vi "流程固件设置对话框.vi"() -> ()   [LabVIEW 2016, in "斯坦道总磷.lvlib"]
uses:
  <vilib>/Utility/miscctls.llb/LVPointTypeDef.ctl
panel:
  in  "修改系列号":bool
  in  "关闭":bool
  in  "外设设置":bool
  in  "固件升级":bool
  in  "流程写入":bool
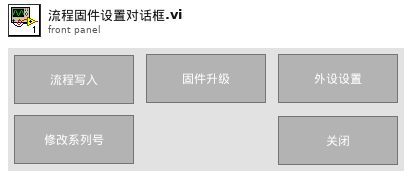
[diagram p1: front panel]
types:
  T1 = typedef "LVPointTypeDef.ctl" = cluster{"Horizontal":i16, "Vertical":i16}
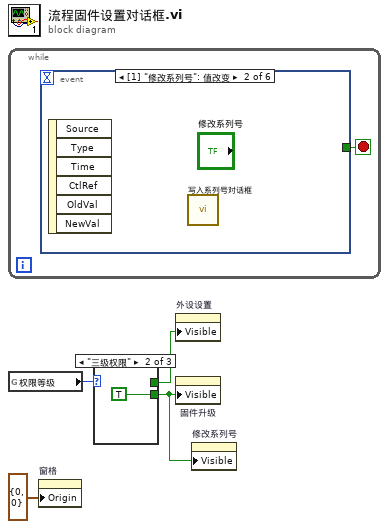
[diagram p0: block diagram]
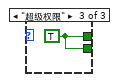
[diagram p3: hidden frame]
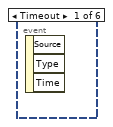
[diagram p4: hidden frame]
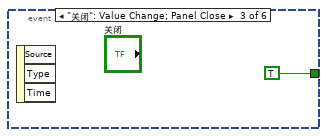
[diagram p5: hidden frame]
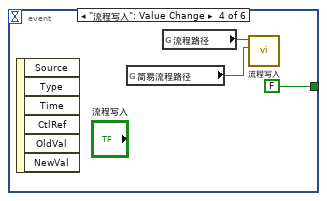
[diagram p6: hidden frame]
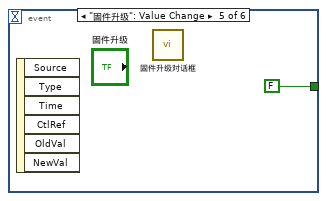
[diagram p7: hidden frame]
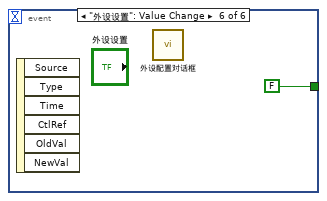
[diagram p8: hidden frame]
diagram:
  n1 = while {
    stop <- w5 stop-if-true
    n2 = event shown="[1] \"修改系列号\": 值改变" {
      selector: _ -> [_ _ _ _ _ _]
      dyn-events: _ -> [_ _ _ _ _ _]
      timeout: _ -> [_ _ _ _ _ _]
      tunnel: [_ _ TRUE FALSE FALSE FALSE] -> w5
      event Timeout {
        n3 = event-data() -> ()  [unwired: 1 in, 3 out]
      }
      event "修改系列号": Value Change {
        n4 = event-data() -> ()  [unwired: 1 in, 6 out]
        n5 = call "写入系列号对话框.vi"() -> ()  [unwired: 12 in]
      }
      event "关闭": Value Change; Panel Close {
        n6 = event-data() -> ()  [unwired: 1 in, 3 out]
      }
      event "流程写入": Value Change {
        n7 = event-data() -> ()  [unwired: 1 in, 6 out]
        n8 = global read "总磷总氮断电保存全局变量.vi" "简易流程路径"() -> (w7:path)
        n9 = global read "总磷总氮断电保存全局变量.vi" "流程路径"() -> (w8:path)
        n10 = call "流程写入.vi"("简易流程路径"=w7, "添加的路径"=w8) -> ()  [unwired: 10 in]
      }
      event "固件升级": Value Change {
        n11 = event-data() -> ()  [unwired: 1 in, 6 out]
        n12 = call "固件升级对话框.vi"() -> ()  [unwired: 12 in]
      }
      event "外设设置": Value Change {
        n13 = event-data() -> ()  [unwired: 1 in, 6 out]
        n14 = call "外设配置对话框.vi"() -> ()  [unwired: 12 in]
      }
    }
  }
  n15 = global read "VAR总磷总氮全局变量.vi" "权限等级"() -> (w3:enum16{"一级权限", "二级权限", "三级权限", "超级权限"})
  n16 = property on="窗格" class="Pane"("Origin"=T1 {"Horizontal"=0, "Vertical"=0} ("原点")) -> ()  [unwired: 2 in, 2 out]
  n17 = case shown="\"三级权限\"" w3 {
    tunnel: [_ TRUE w13] -> w1
    tunnel: [_ _ w13] -> w2
    frame "一级权限", Default {
    }
    frame "三级权限" {
    }
    frame "超级权限" {
      w13 = TRUE
    }
  }
  n18 = property on="外设设置" class="Bool"("Visible"=w2) -> ()  [unwired: 2 in, 2 out]
  n19 = property on="固件升级" class="Bool"("Visible"=w1) -> ()  [unwired: 2 in, 2 out]
  n20 = property on="修改系列号" class="Bool"("Visible"=w1) -> ()  [unwired: 2 in, 2 out]
